vi "Inject Attribute List.vi"(6 "Attributes Ref":refnum<data-value>, 8 "error in (no error)":errorcluster, 11 "Start Spot Free Rinse in":refnum<class "Start Spot Free Rinse.lvclass">) -> (0 "error out":errorcluster, 3 "Start Spot Free Rinse out":refnum<class "Start Spot Free Rinse.lvclass">)   [LabVIEW 2019, in "Start Spot Free Rinse.lvclass"]
uses:
  <vilib>/gpm_packages/@cs/Car-wash/Source/Process Steps/Start Spot Free Rinse/Start Spot Free Rinse.lvclass
  <vilib>/gpm_packages/@cs/lookup-table/Source/LookupTable/LookupTable.lvclass
  <vilib>/gpm_packages/@cs/lookup-table/Source/LookupTable/LookupTable.lvclass/LookupTable.ctl
  <vilib>/gpm_packages/@cs/Car-wash/Source/Process Steps/Start Spot Free Rinse/Start Spot Free Rinse.lvclass/Start Spot Free Rinse.ctl
  67592f74-070b-4603-adf7-90ecc2ff4e90.vi
  <vilib>/gpm_packages/@cs/lookup-table/Source/LookupTable/Read Table Reference.vi
  67592f74-070b-4603-adf7-90ecc2ff4e90.vi/e8f19b0e-b550-4826-a9fd-44a574b76d7d.vi
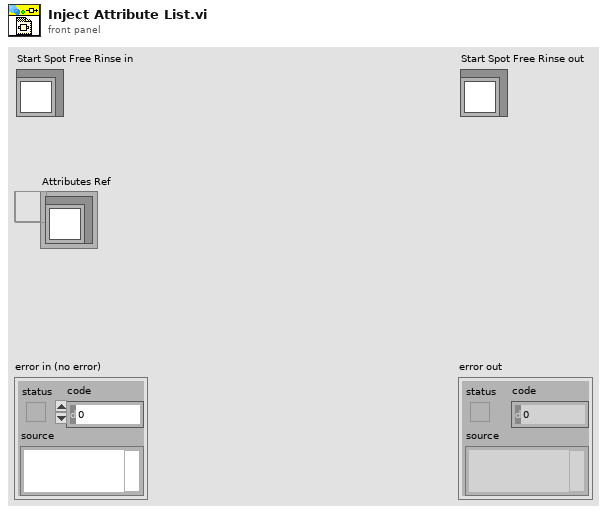
[diagram p1: front panel]
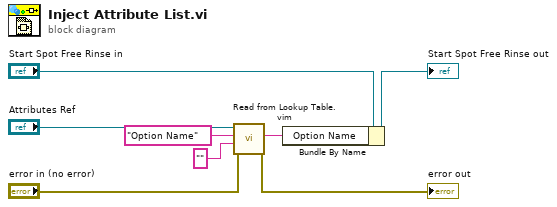
[diagram p0: block diagram]
diagram:
  n1 = call "Read from Lookup Table.vim"("error in (no error)"="error in (no error)", "Type"="", "Item Name"="Option Name", "LookupTable Reference"="Attributes Ref") -> ("error out"=→"error out":errorcluster, "Value"=w6:string)  [unwired: 4 in, 2 out]
  n2 = Bundle By Name(cluster="Start Spot Free Rinse in", "Option Name"=w6) -> (→"Start Spot Free Rinse out":refnum<class "Start Spot Free Rinse.lvclass">)
